vi "Go Back.vi"(8 "error in (no error)":errorcluster, 11 "WebView2 Control in":refnum<class "WebView2 QControl.lvclass">) -> (0 "error out":errorcluster, 3 "WebView2 Control out":refnum<class "WebView2 QControl.lvclass">)   [LabVIEW 2020, in "WebView2 QControl.lvlib" / "WebView2 QControl.lvclass"]
uses:
  WebView2 QControl.lvclass
  WebView2 QControl.lvclass/WebView2 QControl.ctl
  Webview2 Lib/WebView2 Control Object/WebView2 Control.lvclass
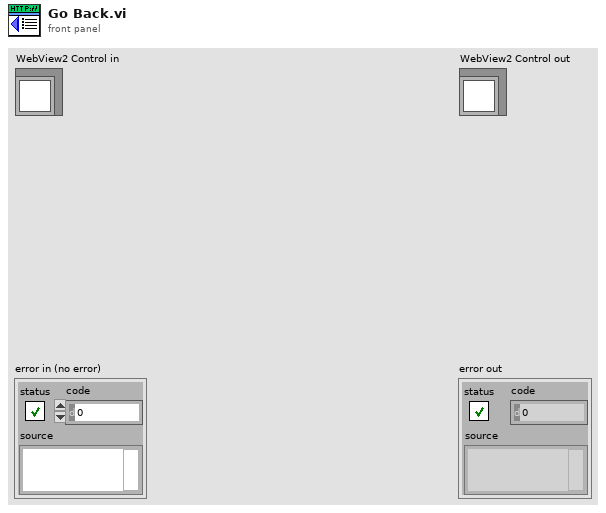
[diagram p1: front panel]
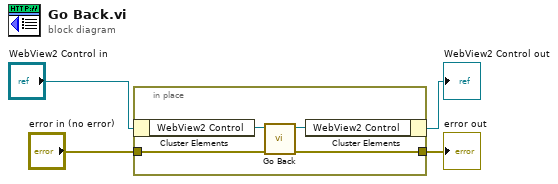
[diagram p0: block diagram]
diagram:
  n1 = in-place {
    in-place-border: "error in (no error)" -> [w8]
    in-place-border: [w7] -> w1
    n2 = in-place-cluster #1("WebView2 Control in") -> ("WebView2 Control"=w6:refnum<class "WebView2 Control.lvclass">)
    n3 = call "Go Back.vi"("error in (no error)"=w8, "WebView2 Control in"=w6) -> ("error out"=w7:errorcluster, "WebView2 Control out"=w5:refnum<class "WebView2 Control.lvclass">)  [unwired: 8 in]
    n4 = in-place-cluster #1("WebView2 Control"=w5) -> (→"WebView2 Control out":refnum<class "WebView2 QControl.lvclass">)
  }
  "error out" <- w1
